vi "lab4.vi"() -> ()   [LabVIEW 2017]
uses:
  <vilib>/addons/Control Design/_Model Construction/Data Typedefs.llb/CD Parametric Time Response Data.ctl
  <vilib>/addons/Control Design/_Model Construction/Special Model Creation.llb/Special Model Creation SubVI/CD Create 1st Order Model.vi
  <vilib>/addons/Control Design/_Model Interconnection/Model Interconnection.llb/Model Interconnection SubVI/cd_Subtract Models (TF and TF).vi
  <vilib>/addons/Control Design/_Dynamic Analysis/Dynamic Analysis.llb/Dynamic Analysis subVI/cd_Stability (Transfer Function).vi
  <vilib>/addons/Control Design/_Dynamic Analysis/Dynamic Analysis.llb/Dynamic Analysis subVI/cd_Pole-Zero Map (Transfer Function).vi
  <vilib>/addons/Control Design/_Utility/Model Viewer.llb/Model Viewer SubVI/cd_Draw Transfer Function Equation (TF).vi
  <vilib>/addons/Control Design/_Time Response Analysis/Time Response.llb/Time Response subVI/cd_Step Response (Transfer Function).vi
  <vilib>/addons/Control Design/_Time Response Analysis/Time Response.llb/Time Response subVI/cd_Parametric Time Response (TF).vi
  <vilib>/addons/Control Design/_Dynamic Analysis/NI_CD_Dynamic Analysis.lvlib
  <vilib>/addons/Control Design/_Utility/NI_CD_Model Viewer.lvlib
  <vilib>/addons/Control Design/_Time Response Analysis/NI_CD_Time Response.lvlib
  <vilib>/addons/Control Design/_Model Construction/NI_CD_Special Model Creation.lvlib
  <vilib>/addons/Control Design/_Model Interconnection/NI_CD_Model Interconnection.lvlib
  <vilib>/addons/Control Design/_Model Construction/NI_LinSys_Data Typedefs.lvlib
panel:
  out "Step Response Graph":cluster{"time":dbl[], dbl[]}[](graph)
  in  "Time Constant (s) 2":dbl format="%.4f"
  in  "Static Gain 2":dbl=1.0 format="%.4f"
  out "Pole-Zero Map":cluster{dbl[], dbl[]}[](graph)
  out "Poles":cdb[](array[numeric]) format="%.2f"
  in  "Tolerance":dbl=1e-08 format="%.2e"
  out "Stability":T1(ring)=enum."undetermined"
  out "Equation":picture
  out "Time Response Parametric Data":T2={"Rise Time (s)"=[[0.0, 0.0], [0.0, 0.0]], "Peak Time (s)"=[[16.01539885840777, 17.159355919722614], [7.372167728473419, 117.70047097528251]], "Settling Time (s)"=[[0.0, 0.0], [0.0, 0.0]], "Overshoot (%)"=[[2.6933680524159342, 1.5395749934973058], [324.8704022191171, -0.0007732741527544107]], "Steady-State Gain"=[[0.0, 0.0], [0.0, 0.0]], "Peak Value"=[[0.0, 0.0], [0.0, 0.0]]}
  out "Time Response":cluster{"time":dbl[], dbl[]}[](graph) caption="Time Response Graph"
  in  "Time Constant (s)":dbl format="%.4f"
  in  "Static Gain":dbl=1.0 format="%.4f"
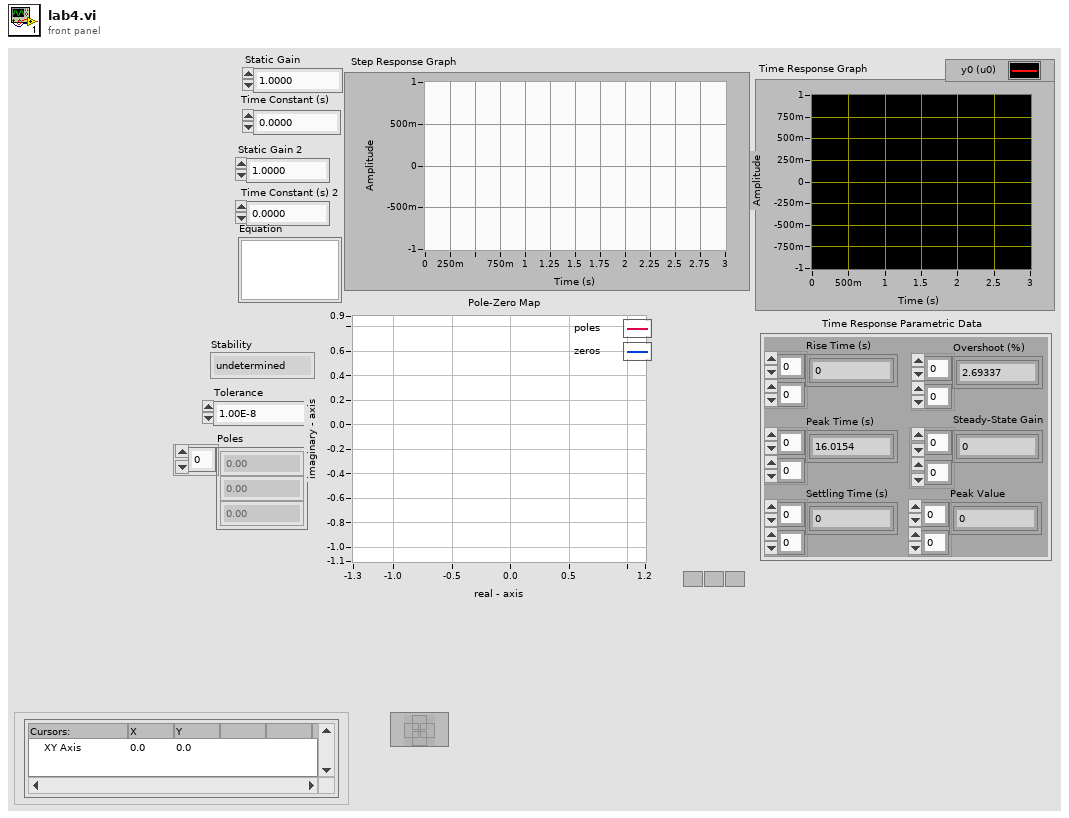
[diagram p1: front panel]
types:
  T1 = enum16{"stable", "marginally stable", "unstable", "undetermined"}
  T2 = typedef "NI_LinSys_Data Typedefs.lvlib/CD Parametric Time Response Data.ctl" = cluster{"Rise Time (s)":dbl[][], "Peak Time (s)":dbl[][], "Settling Time (s)":dbl[][], "Overshoot (%)":dbl[][], "Steady-State Gain":dbl[][], "Peak Value":dbl[][]}
  T3 = typedef "NI_LinSys_Model Typedefs.lvlib/CD Transfer Function Model (MIMO).ctl" = cluster{"properties":T4, "transfer function(s)":T5[][]}
  T4 = typedef "NI_LinSys_Model Typedefs.lvlib/CD General Elements.ctl" = cluster{"Model name":string, "Input names":string[], "Output names":string[], "Input Delays":dbl[], "Output Delays":dbl[], "Sampling Time":dbl, "Notes":string}
  T5 = typedef "NI_LinSys_Model Typedefs.lvlib/CD Transfer Function Model (SISO).ctl" = cluster{"Numerator":dbl[], "Denominator":dbl[], "delay":dbl}
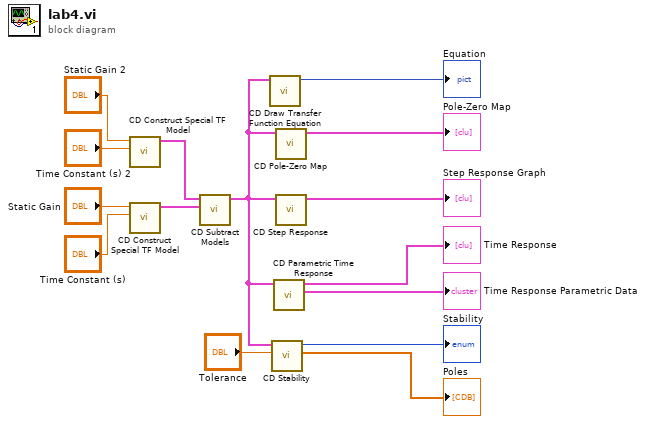
[diagram p0: block diagram]
diagram:
  n1 = call-poly <vilib>:"CD Construct Special TF Model.vi"("Time Constant (s)"="Time Constant (s) 2", "Static Gain"="Static Gain 2") -> ("Transfer Function Model"=w3:T3)  [unwired: 8 in, 1 out]
  n2 = call-poly <vilib>:"CD Construct Special TF Model.vi"("Time Constant (s)"="Time Constant (s)", "Static Gain"="Static Gain") -> ("Transfer Function Model"=w2:T3)  [unwired: 8 in, 1 out]
  n3 = call-poly <vilib>:"CD Subtract Models.vi"("Model 2"=w2, "Model 1"=w3) -> ("Model out"=w4:T3)  [unwired: 8 in, 1 out]
  n4 = call-poly <vilib>:"CD Draw Transfer Function Equation.vi"("Transfer Function Model"=w4) -> ("Equation"=→"Equation":picture)  [unwired: 8 in, 2 out]
  n5 = call-poly <vilib>:"CD Stability.vi"("Tolerance"="Tolerance", "Transfer Function Model"=w4) -> ("Poles"=→"Poles":cdb[], "Stability"=→"Stability":T1)  [unwired: 7 in, 1 out]
  n6 = call-poly <vilib>:"CD Parametric Time Response.vi"("Transfer Function Model"=w4) -> ("Time Response Parametric Data"=→"Time Response Parametric Data":T2, "Time Response"=→"Time Response":cluster{"time":dbl[], dbl[]}[])  [unwired: 7 in, 2 out]
  n7 = call-poly <vilib>:"CD Pole-Zero Map.vi"("Transfer Function Model"=w4) -> ("Pole-Zero Map"=→"Pole-Zero Map":cluster{dbl[], dbl[]}[])  [unwired: 7 in, 3 out]
  n8 = call-poly <vilib>:"CD Step Response.vi"("Transfer Function Model"=w4) -> ("Step Response Graph"=→"Step Response Graph":cluster{"time":dbl[], dbl[]}[])  [unwired: 8 in, 2 out]
